vi "Exp_CCD_SetAcdSpeed.vi"(8 "error in (no error)":errorcluster, 10 "Speed (MHz)":dbl, 11 "LightField Automation in":refnum<class "LightField Automation.lvclass">) -> (0 "error out":errorcluster, 3 "LightField Automation out":refnum<class "LightField Automation.lvclass">)   [LabVIEW 2015, in "LightField Automation.lvclass"]
uses:
  LightField Automation.lvclass
  C:/Program Files/Princeton Instruments/LightField/PrincetonInstruments.LightFieldAddInSupportServices.dll
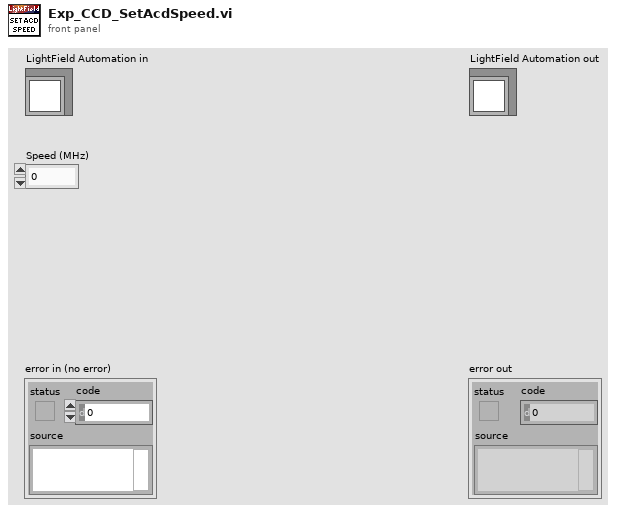
[diagram p1: front panel]
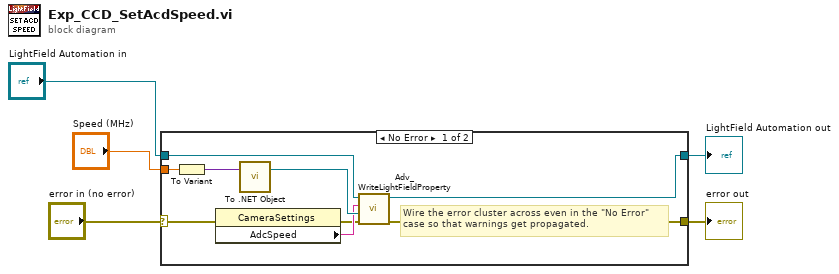
[diagram p0: block diagram]
diagram:
  n1 = case shown="No Error" "error in (no error)" {
    selector: "error in (no error)" -> [w7 w16]
    tunnel: [w6 w16] -> w4
    tunnel: [w9 w15] -> w2
    tunnel: "LightField Automation in" -> [w10 w15]
    tunnel: "Speed (MHz)" -> [w13 _]
    frame No Error {
      # "Wire the error cluster across even in the \"No Error\"\ncase so that warnings get propagated."
      n2 = To Variant(anything=w13) -> (Variant=w14:variant)
      n3 = property class="CameraSettings"(error in=w7) -> (error out=w8:errorcluster, "AdcSpeed"=w11:string)  [unwired: 1 in, 1 out]
      n4 = call <vilib>:"To .NET Object.vi"("anything"=w14) -> (".NET object"=w12:refnum<k24>)  [unwired: 1 in, 1 out]
      n5 = call "Adv_WriteLightFieldProperty.vi"("error in (no error)"=w8, "value"=w12, "setting"=w11, "LightField Automation in"=w10) -> ("error out"=w6:errorcluster, "LightField Automation out"=w9:refnum<class "LightField Automation.lvclass">)  [unwired: 6 in]
    }
    frame Error {
    }
  }
  "error out" <- w4
  "LightField Automation out" <- w2
